vi "Float Encoder.vi"(9 "Array In":u8[](array[numeric]), 10 "Key":u32, 11 "Value":sgl) -> (1 "Array":u8[](array[numeric]))   [LabVIEW 2018]
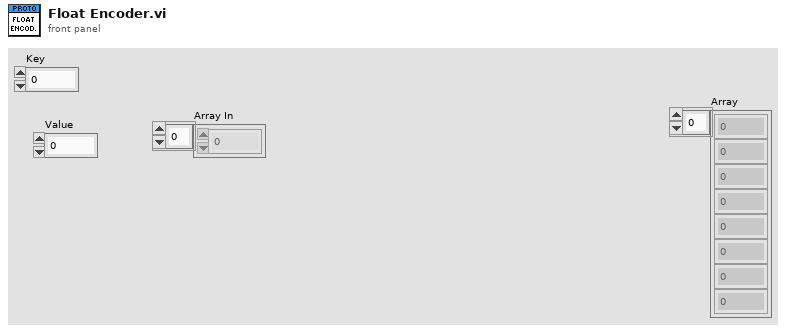
[diagram p1: front panel]
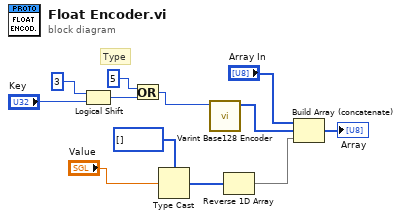
[diagram p0: block diagram]
diagram:
  # "Type"
  n1 = Logical Shift(y=i16 3, x="Key") -> (x << y=w10:u32)
  n2 = Or(x=u32 5, y=w10) -> (x .or. y?=w8:u32)
  n3 = Type Cast(type=u8[] [], x="Value") -> (*(type *) &x=w2:u8[])
  n4 = call "Varint Base128 Encoder.vi"("Numeric"=w8) -> ("Array"=w7:u8[])  [unwired: 10 in]
  n5 = Reverse 1D Array(array=w2) -> (reversed array=w1:u8[])
  n6 = Build Array (concatenate)("Array In", w7, w1) -> (→"Array":u8[])
